vi "Extract LV Icon Data.vi"(8 "error in (no error)":errorcluster, 10 "LabVIEW Icon in (original)":string, 11 "Data in":T1={"Class"={"Ants"=refnum, "Layer"=refnum, "Templates"=refnum, "Icon"=refnum, "Glyph"=refnum, "Settings"=refnum, "Tools"=refnum}, "Ref"={"Add Layer"=refnum, "Remove Layer"=refnum, "Line Text"=[], "Body Text Spec"=refnum, "DNL_Font"=refnum, "glyph path str"=refnum, "templates path str"=refnum, "Arrow Up"=refnum, "Arrow Down"=refnum, "IE VI Ref"=refnum, "Glyphs tree"=refnum, "Templates tree"=refnum, "Layer Icon Text"=refnum, "Layer Template"=refnum, "Body Text"=refnum, "Search Templates"=refnum, "TextMarker"=refnum, "Tab Control"=refnum, "Search Glyphs"=refnum, "Line Color"=refnum, "DNL_Glyphs []"=refnum, "Fill Color"=refnum, "Tools"=refnum, "Icon"=refnum, "Preview"=refnum, "Ants"=refnum, "Terminals"=refnum, "menu reference"=refnum, "LayerNames"=[], "GlyphLoadAnimation"=refnum, "TemplateLoadAnimation"=refnum, "refreshGlyphs"=refnum, "refreshTemplates"=refnum}, "Support"={"AntsRect"={"left"=0, "top"=0, "right"=0, "bottom"=0}, "Mouse Move Coords"={"Horizontal"=0, "Vertical"=0}, "Mouse Down Coords"={"Horizontal"=0, "Vertical"=0}, "Temp Coord"={"Horizontal"=0, "Vertical"=0}, "Action"=enum."Default", "Edge Color"=4914962, "Fill Color"=16860, "Mouse Down?"=FALSE, "Draft Mode?"=FALSE, "Temp Icon"=bytes[3102], "CTRL Pressed"=FALSE, "Move Selection?"=FALSE, "AntsRect Orig"={"left"=0, "top"=0, "right"=0, "bottom"=0}, "Text"="", "TM Set?"=FALSE, "Mouse inside icon?"=FALSE, "Tool (old value)"=0, "Pencil Move Color"=0, "Swap Colors?"=FALSE, "Shift pressed?"=FALSE}}) -> (0 "error out":errorcluster, 2 "LabVIEW Icon out":string, 3 "Data out":T1={"Class"={"Ants"=refnum, "Layer"=refnum, "Templates"=refnum, "Icon"=refnum, "Glyph"=refnum, "Settings"=refnum, "Tools"=refnum}, "Ref"={"Add Layer"=refnum, "Remove Layer"=refnum, "Line Text"=[], "Body Text Spec"=refnum, "DNL_Font"=refnum, "glyph path str"=refnum, "templates path str"=refnum, "Arrow Up"=refnum, "Arrow Down"=refnum, "IE VI Ref"=refnum, "Glyphs tree"=refnum, "Templates tree"=refnum, "Layer Icon Text"=refnum, "Layer Template"=refnum, "Body Text"=refnum, "Search Templates"=refnum, "TextMarker"=refnum, "Tab Control"=refnum, "Search Glyphs"=refnum, "Line Color"=refnum, "DNL_Glyphs []"=refnum, "Fill Color"=refnum, "Tools"=refnum, "Icon"=refnum, "Preview"=refnum, "Ants"=refnum, "Terminals"=refnum, "menu reference"=refnum, "LayerNames"=[], "GlyphLoadAnimation"=refnum, "TemplateLoadAnimation"=refnum, "refreshGlyphs"=refnum, "refreshTemplates"=refnum}, "Support"={"AntsRect"={"left"=0, "top"=0, "right"=0, "bottom"=0}, "Mouse Move Coords"={"Horizontal"=0, "Vertical"=0}, "Mouse Down Coords"={"Horizontal"=0, "Vertical"=0}, "Temp Coord"={"Horizontal"=0, "Vertical"=0}, "Action"=enum."Default", "Edge Color"=4914962, "Fill Color"=16860, "Mouse Down?"=FALSE, "Draft Mode?"=FALSE, "Temp Icon"=bytes[3102], "CTRL Pressed"=FALSE, "Move Selection?"=FALSE, "AntsRect Orig"={"left"=0, "top"=0, "right"=0, "bottom"=0}, "Text"="", "TM Set?"=FALSE, "Mouse inside icon?"=FALSE, "Tool (old value)"=0, "Pencil Move Color"=0, "Swap Colors?"=FALSE, "Shift pressed?"=FALSE}})   [LabVIEW 2020]
uses:
  Class/Ants/Ants.lvclass
  Class/FakedArray/FakedArray.lvclass
  vi.lib/LabVIEW Icon API/lv_icon/Classes/Icon/Icon.lvclass
  Class/Icon Library/Glyph.lvclass
  Class/Settings/Settings.lvclass
  Class/Tools/Tools Paint.lvclass
  <vilib>/Utility/miscctls.llb/LVPoint32TypeDef.ctl
  Controls/SupportClass_Action.ctl
  vi.lib/LabVIEW Icon API/lv_icon/Controls/IEColor.ctl
  Controls/SupportClass.ctl
  Controls/References Cluster.ctl
  vi.lib/LabVIEW Icon API/lv_icon/lv_icon.lvlib
  Controls/IE Classes.ctl
  Controls/Global Data.ctl
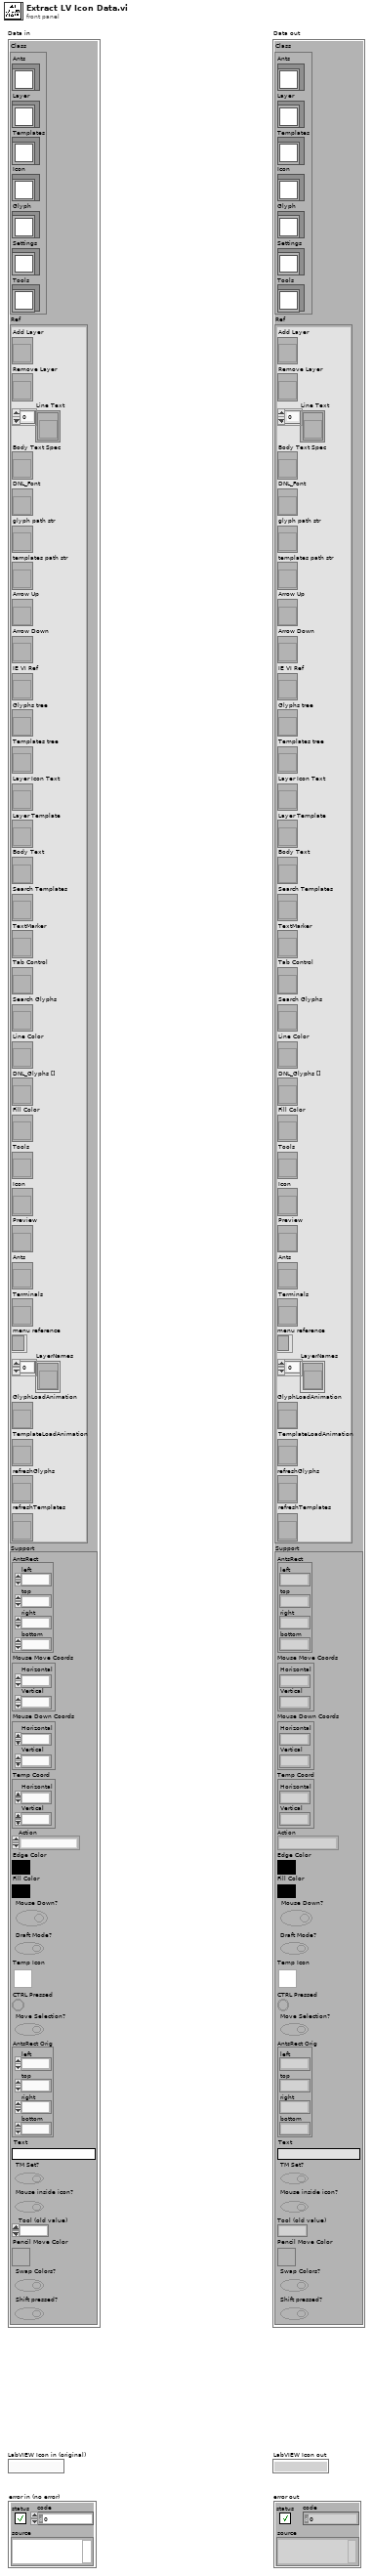
[diagram p1: front panel]
types:
  T1 = typedef "lv_icon.lvlib/Global Data.ctl" = cluster{"Class":T2, "Ref":T3, "Support":T4}
  T2 = typedef "IE Classes.ctl" = cluster{"Ants":refnum<class "Ants.lvclass">, "Layer":refnum<class "FakedArray.lvclass">, "Templates":refnum<class "FakedArray.lvclass">, "Icon":refnum<class "Icon.lvclass">, "Glyph":refnum<class "Glyph.lvclass">, "Settings":refnum<class "Settings.lvclass">, "Tools":refnum<class "Tools Paint.lvclass">}
  T3 = typedef "lv_icon.lvlib/References Cluster.ctl" = cluster{"Add Layer":refnum<vi>, "Remove Layer":refnum<vi>, "Line Text":refnum<vi>[], "Body Text Spec":refnum<vi>, "DNL_Font":refnum<vi>, "glyph path str":refnum<vi>, "templates path str":refnum<vi>, "Arrow Up":refnum<vi>, "Arrow Down":refnum<vi>, "IE VI Ref":refnum<vi>, "Glyphs tree":refnum<vi>, "Templates tree":refnum<vi>, "Layer Icon Text":refnum<vi>, "Layer Template":refnum<vi>, "Body Text":refnum<vi>, "Search Templates":refnum<vi>, "TextMarker":refnum<vi>, "Tab Control":refnum<vi>, "Search Glyphs":refnum<vi>, "Line Color":refnum<vi>, "DNL_Glyphs []":refnum<vi>, "Fill Color":refnum<vi>, "Tools":refnum<vi>, "Icon":refnum<vi>, "Preview":refnum<vi>, "Ants":refnum<vi>, "Terminals":refnum<vi>, "menu reference":refnum<k9>, "LayerNames":refnum<vi>[], "GlyphLoadAnimation":refnum<vi>, "TemplateLoadAnimation":refnum<vi>, "refreshGlyphs":refnum<vi>, "refreshTemplates":refnum<vi>}
  T4 = typedef "SupportClass.ctl" = cluster{"AntsRect":cluster{"left":i16, "top":i16, "right":i16, "bottom":i16}, "Mouse Move Coords":T5, "Mouse Down Coords":T5, "Temp Coord":T5, "Action":T6, "Edge Color":T7, "Fill Color":T7, "Mouse Down?":bool, "Draft Mode?":bool, "Temp Icon":picture, "CTRL Pressed":bool, "Move Selection?":bool, "AntsRect Orig":cluster{"left":i16, "top":i16, "right":i16, "bottom":i16}, "Text":string, "TM Set?":bool, "Mouse inside icon?":bool, "Tool (old value)":u32, "Pencil Move Color":u32, "Swap Colors?":bool, "Shift pressed?":bool}
  T5 = typedef "LVPoint32TypeDef.ctl" = cluster{"Horizontal":i32, "Vertical":i32}
  T6 = typedef "SupportClass_Action.ctl" = enum16{"Default", "Move Selection", "Glyph Library", "Tool"}
  T7 = typedef "IEColor.ctl" = u32
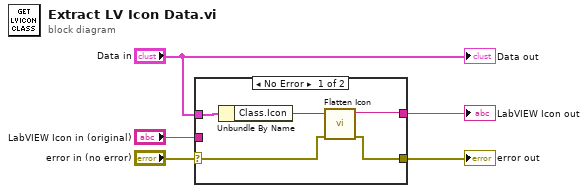
[diagram p0: block diagram]
diagram:
  n1 = case shown="No Error" "error in (no error)" {
    selector: "error in (no error)" -> [w7 w12]
    tunnel: [w8 w11] -> w1
    tunnel: "Data in" -> [w10 _]
    tunnel: [w6 w12] -> w3
    tunnel: "LabVIEW Icon in (original)" -> [_ w11]
    frame No Error {
      n2 = Unbundle By Name(w10) -> ("Class.Icon"=w9:refnum<class "Icon.lvclass">)
      n3 = call "Flatten Icon.vi"("Error In"=w7, "Icon"=w9) -> ("Error Out"=w6:errorcluster, "String"=w8:string)  [unwired: 8 in]
    }
    frame Error {
    }
  }
  "error out" <- w3
  "LabVIEW Icon out" <- w1
  "Data out" <- "Data in"
